vi "vecProj.vi"(2 "error in (no error)":errorcluster, 3 "N":i32, 4 "th_min":T1, 5 "th":T1, 6 "th_max":T1, 7 "a":T1) -> (0 "error out":errorcluster, 1 "Proj_th (a)":T1)   [LabVIEW 2021]
uses:
  <vilib>/Analysis/Matrix/Datatypes/RealMatrix.ctl
  <vilib>/Analysis/Matrix/NI_Matrix.lvlib
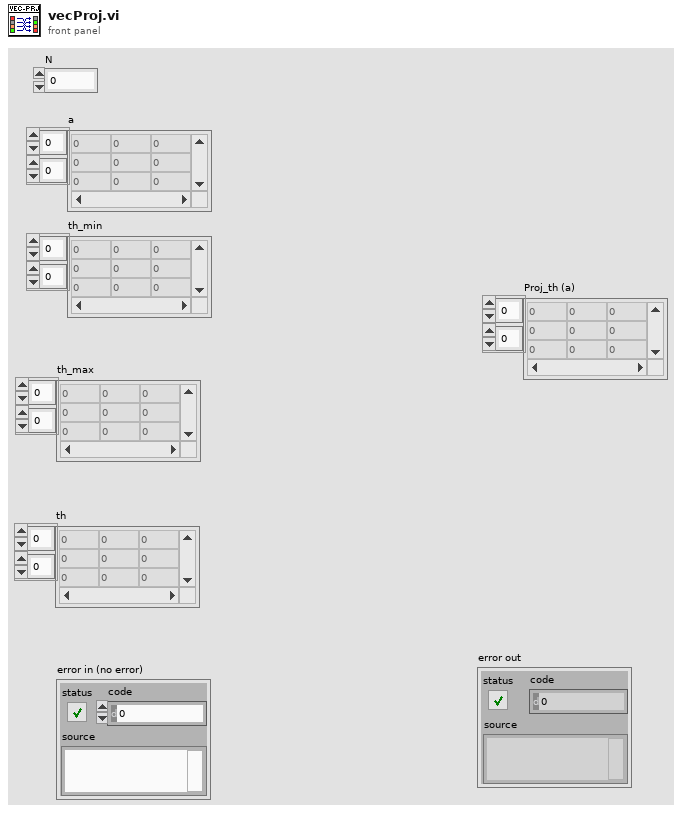
[diagram p1: front panel]
types:
  T1 = typedef "NI_Matrix.lvlib/RealMatrix.ctl" = dbl[][]
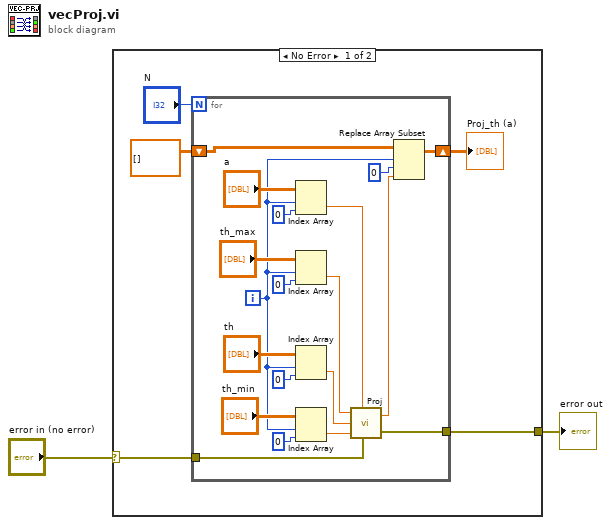
[diagram p0: block diagram]
diagram:
  n1 = case shown="No Error" "error in (no error)" {
    selector: "error in (no error)" -> [w4 w27]
    tunnel: [w3 w27] -> w1
    frame No Error {
      n2 = for {
        N: "N" -> [_]
        shift-right: [w12] -> w6
        shift-left: T1 [] ("Real Matrix") -> [w13]
        tunnel: w4 -> [w11]
        tunnel: [w10] -> w3
        i -> [w9]
        n3 = Index Array(array="a", index (row)=w9, index (col)=0) -> (element=w16:dbl)
        n4 = Index Array(array="th_max", index (row)=w9, index (col)=0) -> (element=w18:dbl)
        n5 = Index Array(array="th", index (row)=w9, index (col)=0) -> (element=w21:dbl)
        n6 = Index Array(array="th_min", index (row)=w9, index (col)=0) -> (element=w24:dbl)
        n7 = call "Proj.vi"("th_max"=w18, "a"=w16, "th"=w21, "th_min"=w24, "error in (no error)"=w11) -> ("Proj_th (a)"=w15:dbl, "error out"=w10:errorcluster)
        n8 = Replace Array Subset(array=w13, new element=w15, index (row)=w9, index (col)=0 ("disabled index (col)")) -> (w12:T1)
      }
      "Proj_th (a)" <- w6
    }
    frame Error {
    }
  }
  "error out" <- w1
